vi "FTW-TestExecutive-LoadSequence.vi"(0 "FTW Actor Connector In":refnum<class "FTW-ActorConnector.lvclass">, 7 "Sequence":string, 11 "error in (no error)":errorcluster) -> (4 "FTW Actor Connector":refnum<class "FTW-ActorConnector.lvclass">, 8 "Loaded Sequence":T1[](array[typedef]) {"Results"."Start Time" format="%<%Y-%m-%d %H:%M:%S%03u>T"; "Results"."Elapsed Time" format="%<%H:%M:%S%3u>t"; "Elapsed Time" format="%<%H:%M:%S%3u>t"}, 14 "Roundtrip Time":dbl format="%.6f sec", 15 "error out":errorcluster)   [LabVIEW 2018]
uses:
  Connector/FTW-ActorConnector.lvclass
  FTW-TestExecutive-Step.ctl
  FTW-TestExecutive-Step-State.ctl
  FTW-TestExecutive-Results.ctl
  27caabc6-e458-4741-81bd-9b28765e690e.vi
  JSON/core/FTW-JSON-Core-EncodingFlags.vi
  Reflection/FTW-Reflection-Type.vi
  JSON/FTW-JSON-Parse.vi
  container/FTW-Container-GetFlattenedValue.vi
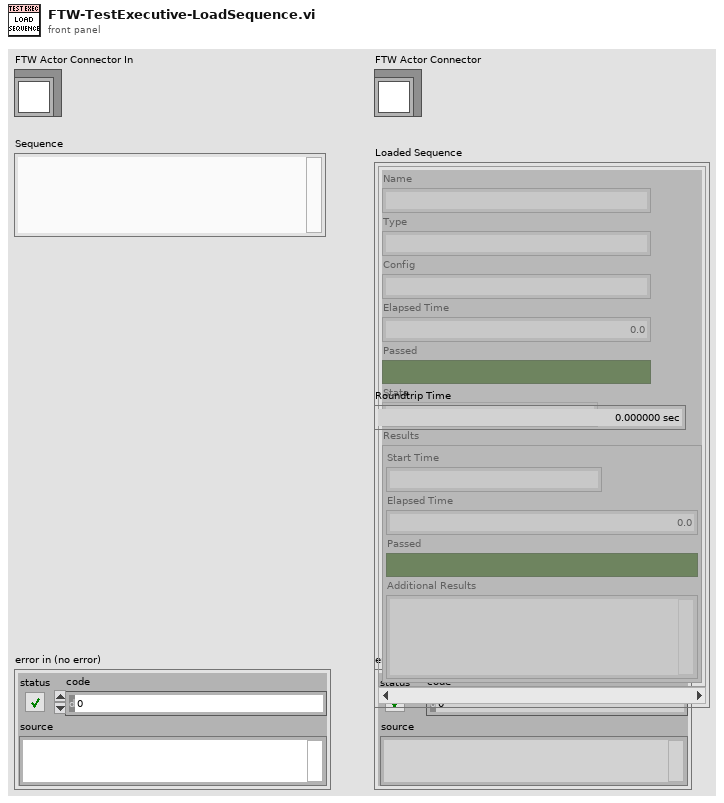
[diagram p1: front panel]
types:
  T1 = typedef "FTW-TestExecutive-Step.ctl" = cluster{"Name":string, "Type":string, "Config":string, "Elapsed Time":dbl, "Passed":bool, "State":T2, "Results":T3}
  T2 = typedef "FTW-TestExecutive-Step-State.ctl" = enum8{"None", "Failed", "Passed", "Timed out", "Aborted"}
  T3 = typedef "FTW-TestExecutive-Results.ctl" = cluster{"Start Time":timestamp, "Elapsed Time":dbl, "Passed":bool, "Additional Results":string}
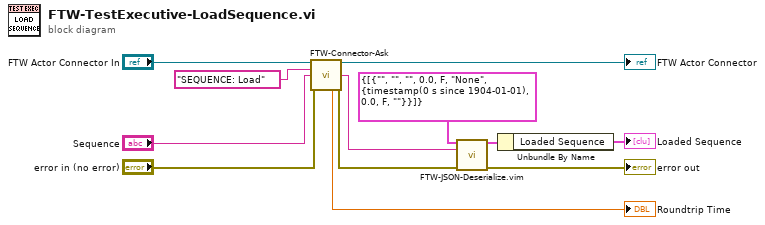
[diagram p0: block diagram]
diagram:
  n1 = call "FTW-Connector-Ask.vi"("FTW Actor Connector"="FTW Actor Connector In", "Request Header"="SEQUENCE: Load", "Request Body"="Sequence", "error in"="error in (no error)") -> ("FTW Actor Connector out"=→"FTW Actor Connector":refnum<class "FTW-ActorConnector.lvclass">, "Response Body"=w5:string, "Roundtrip Time"=→"Roundtrip Time":dbl, "error out"=w8:errorcluster)  [unwired: 6 in, 2 out]
  n2 = call "FTW-JSON-Deserialize.vim"("Type In"=cluster{"Loaded Sequence":T1[]} {"Loaded Sequence"=[{"Name"="", "Type"="", "Config"="", "Elapsed Time"=0.0, "Passed"=FALSE, "State"=enum."None", "Results"={"Start Time"=timestamp(0 s since 1904-01-01), "Elapsed Time"=0.0, "Passed"=FALSE, "Additional Results"=""}}]}, "JSON String"=w5, "error in"=w8) -> ("Type Out"=w3:cluster{"Loaded Sequence":T1[]}, "error out"=→"error out":errorcluster)  [unwired: 11 in]
  n3 = Unbundle By Name(w3) -> ("Loaded Sequence"=→"Loaded Sequence":T1[])
